vi "q4 inc dec counter.vi"() -> ()   [LabVIEW 2025]
panel:
  in  "stop":bool
  out "count = 0":bool
  out "count":dbl
  in  "decrement":bool
  in  "increment":bool
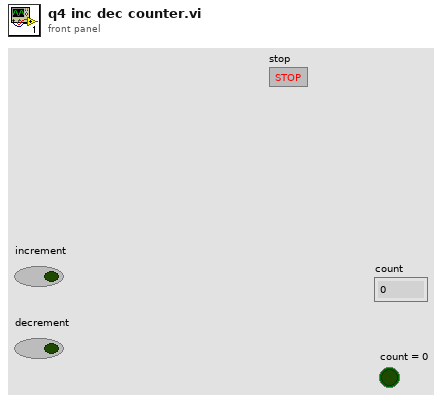
[diagram p1: front panel]
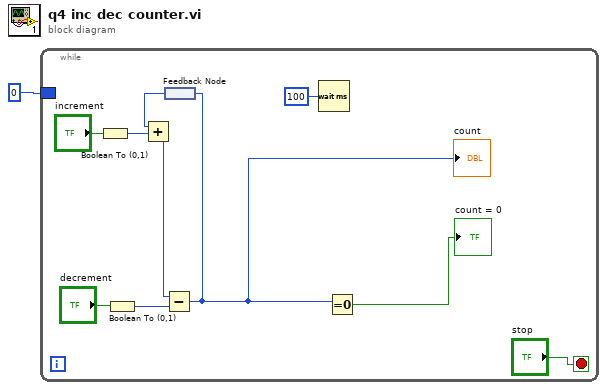
[diagram p0: block diagram]
diagram:
  n1 = while {
    border: 0 -> [_]
    stop <- "stop" stop-if-true
    n2 = Boolean To (0,1)(Boolean="increment") -> (0, 1=w9:i16)
    n3 = Boolean To (0,1)(Boolean="decrement") -> (0, 1=w7:i16)
    n4 = feedback #1() -> (w8:i32)
    n5 = Add(x=w8, y=w9) -> (x+y=w6:i32)
    n6 = Subtract(x=w6, y=w7) -> (x-y=w5:i32)
    "count" <- w5
    n7 = feedback-in #1(w5) -> ()
    n8 = Wait (ms)(milliseconds to wait=100) -> ()  [unwired: 1 out]
    n9 = Equal To 0?(x=w5) -> (x = 0?=→"count = 0":bool)
  }
